vi "Check is Upgrade Request.vi"(11 "Request in":refnum<class "Request.lvclass">) -> (0 "error out":errorcluster, 1 "Upgrade Request?":bool, 2 "Sec-WebSocket-Version":string, 3 "Sec-WebSocket-Key":string)   [LabVIEW 2020, in "Stream-Websocket.lvlib"]
uses:
  Stream-Websocket.lvlib
  <vilib>/IlluminatedG/IG HTTP Utils/HTTP Utils/Request/Request.lvclass
  <vilib>/IlluminatedG/IG HTTP Utils/HTTP Utils/Method.ctl
  <vilib>/IlluminatedG/IG HTTP Utils/HTTP Utils/HTTP Utils.lvlib
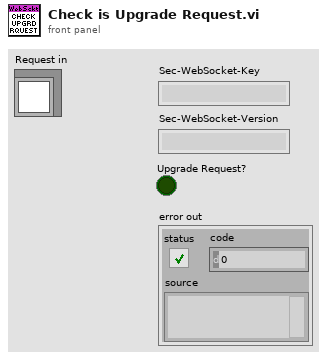
[diagram p1: front panel]
types:
  T1 = typedef "HTTP Utils.lvlib/Method.ctl" = enum16{"GET", "HEAD", "POST", "PUT", "DELETE", "CONNECT", "OPTIONS", "TRACE", "PATCH"}
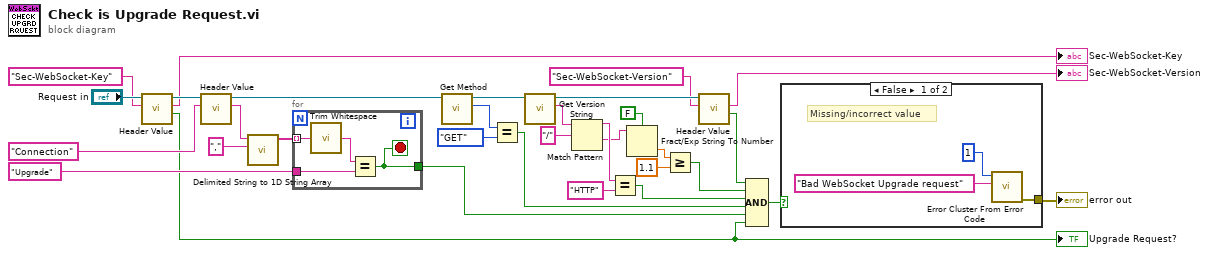
[diagram p0: block diagram]
diagram:
  n1 = call <vilib>:"Header Value.vi"("Header"="Sec-WebSocket-Key", "Request in"="Request in") -> ("Exists"=w7:bool, "Value"=→"Sec-WebSocket-Key":string, "Request out"=w30:refnum<class "Request.lvclass">)  [unwired: 6 in, 1 out]
  "Upgrade Request?" <- w7
  n2 = call <vilib>:"Header Value.vi"("Header"="Connection", "Request in"=w30) -> ("Value"=w3:string, "Request out"=w25:refnum<class "Request.lvclass">)  [unwired: 6 in, 2 out]
  n3 = call <vilib>:"Delimited String to 1D String Array.vi"("delimiter"=",", "delimited string"=w3) -> ("string array"=w1:string[])  [unwired: 9 in]
  n4 = for {
    tunnel: "Upgrade" -> [w36]
    tunnel: [w33] -> w26
    tunnel: w1 -> [w35] mode=indexing
    stop <- w33 stop-if-true
    n5 = call <vilib>:"Trim Whitespace.vi"("string"=w35) -> ("trimmed string"=w34:string)  [unwired: 1 in]
    n6 = Equal?(x=w34, y=w36) -> (x = y?=w33:bool)
  }
  n7 = call <vilib>:"Get Method.vi"("Request in"=w25) -> ("Method"=w24:T1, "Request out"=w22:refnum<class "Request.lvclass">)  [unwired: 8 in, 1 out]
  n8 = Equal?(x=w24, y=Method."GET") -> (x = y?=w21:bool)
  n9 = call <vilib>:"Get Version String.vi"("Request in"=w22) -> ("Version String"=w20:string, "Request out"=w11:refnum<class "Request.lvclass">)  [unwired: 8 in, 1 out]
  n10 = Match Pattern(string=w20, regular expression="/") -> (before substring=w18:string, after substring=w16:string)  [unwired: 1 in, 2 out]
  n11 = Equal?(x=w18, y="HTTP") -> (x = y?=w14:bool)
  n12 = Fract/Exp String To Number(use system decimal point (T)=FALSE, string=w16) -> (number=w15:dbl)  [unwired: 2 in, 1 out]
  n13 = Greater Or Equal?(x=w15, y=1.1) -> (x >= y?=w12:bool)
  n14 = call <vilib>:"Header Value.vi"("Header"="Sec-WebSocket-Version", "Request in"=w11) -> ("Exists"=w8:bool, "Value"=→"Sec-WebSocket-Version":string)  [unwired: 6 in, 2 out]
  n15 = Compound Arithmetic op=AND(w8, w12, w14, w21, w26, w7) -> (w6:bool)
  n16 = case shown="False" w6 {
    tunnel: [w37 _] -> w5
    frame False {
      # "Missing/incorrect value"
      n17 = call <vilib>:"Error Cluster From Error Code.vi"("error message (\"\")"="Bad WebSocket Upgrade request" ("error message (\"\")"), "error code (0)"=1) -> ("error out"=w37:errorcluster)  [unwired: 7 in]
    }
    frame True {
      # "Good request"
    }
  }
  "error out" <- w5
